vi "DefaultFromIni.vi"(8 "error in (no error)":errorcluster, 11 "SyncPlugin":refnum<class "SyncPluginBase.lvclass">) -> (0 "error out":errorcluster, 3 "SyncPlugin":refnum<class "SyncPluginBase.lvclass">)   [LabVIEW 2014, in "SyncPlugins.lvlib" / "SyncPluginBase.lvclass"]
uses:
  SyncPluginBase.lvclass
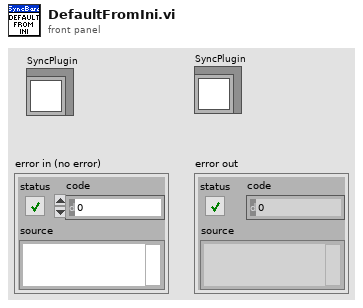
[diagram p1: front panel]
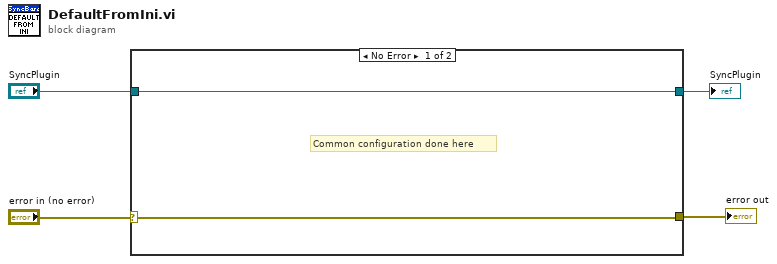
[diagram p0: block diagram]
diagram:
  n1 = case shown="No Error" "error in (no error)" {
    selector: "error in (no error)" -> [w6 w8]
    tunnel: [w6 w8] -> w3
    tunnel: [w5 w7] -> w2
    tunnel: "SyncPlugin" -> [w5 w7]
    frame No Error {
      # "Common configuration done here"
    }
    frame Error {
    }
  }
  "SyncPlugin" <- w2
  "error out" <- w3
